vi "封面.vi"() -> ()   [LabVIEW 2013]
uses:
  <vilib>/Utility/config.llb/Config Data RefNum.ctl
  <vilib>/Utility/config.llb/NI_LVConfig.lvlib
panel:
  in  "版本":string
  in  "编号":string
  in  "封面表":T1
  in  "stop":bool
  # "油动机试验报告\nACTUATOR TEST REPORT"
  # "上海汽轮机厂\nSHANGHAI TURBINE PLANT"
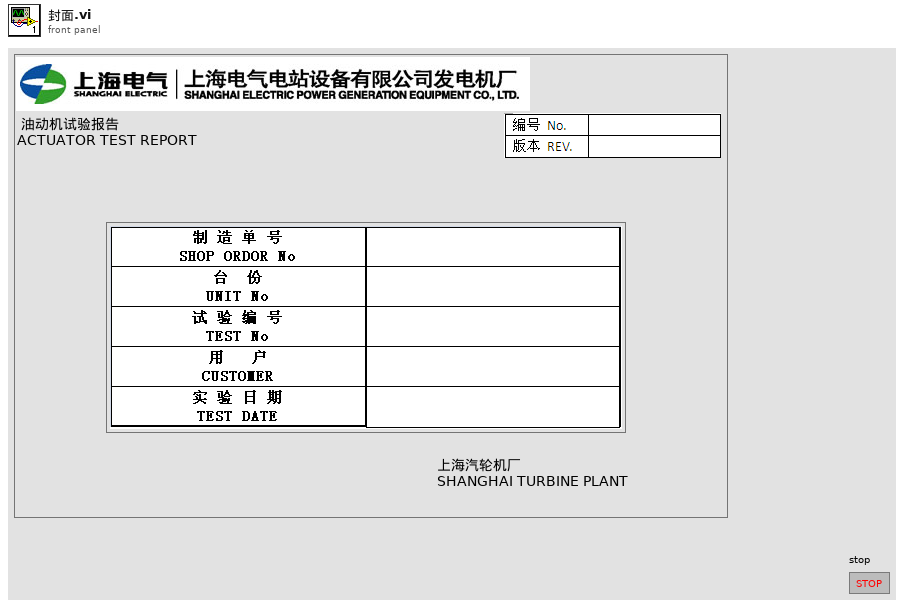
[diagram p1: front panel]
types:
  T1 = typedef "封面表.ctl" = cluster{"制造单号":string, "台份":string, "试验编号":string, "用户":string, "试验日期":string}
  T2 = typedef "NI_LVConfig.lvlib/Config Data RefNum.ctl" = refnum<k1>
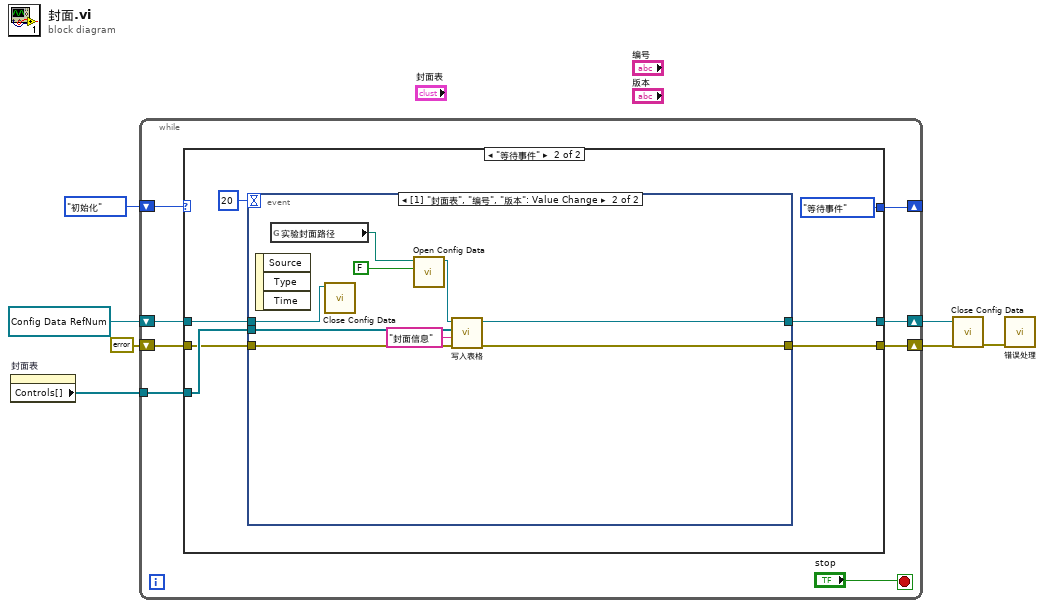
[diagram p0: block diagram]
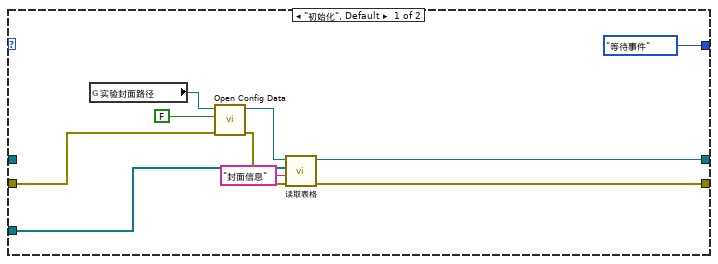
[diagram p2: hidden frame]
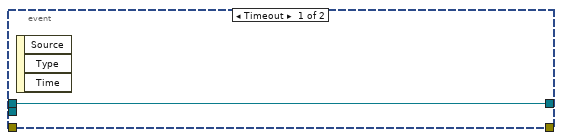
[diagram p3: hidden frame]
diagram:
  w6 = T2 refnum items=["config data"] ("引用句柄输入")
  n1 = property on="封面表" class="Clust (strict)"() -> ("Controls[]"=w5:refnum<vi>[])  [unwired: 2 in, 2 out]
  n2 = while {
    shift-right: [w13] -> _
    shift-left: enum16{"初始化", "等待事件"}."初始化" -> [w14]
    shift-right: [w12] -> w4
    shift-left: w6 -> [w10]
    tunnel: w5 -> [w11]
    shift-right: [w9] -> w3
    shift-left: errorcluster {"status"=FALSE, "code"=0, "source"=""} ("错误输出") -> [w8]
    stop <- "stop" stop-if-true
    n3 = case shown="\"等待事件\"" w14 {
      tunnel: [enum16{"初始化", "等待事件"}."等待事件" enum16{"初始化", "等待事件"}."等待事件"] -> w13
      tunnel: [w22 w28] -> w12
      tunnel: w11 -> [w21 w30]
      tunnel: w10 -> [_ w29]
      tunnel: [w20 w27] -> w9
      tunnel: w8 -> [w18 w26]
      frame "初始化", Default {
        n4 = global read "实验封面路径.vi" "实验封面路径"() -> (w17:path)
        n5 = call <vilib>:"Open Config Data.vi"("error in (no error)"=w18, "create file if necessary (T)"=FALSE, "configuration file path"=w17) -> ("error out"=w19:errorcluster, "refnum"=w24:T2)  [unwired: 6 in, 1 out]
        n6 = call "读取表格.vi"("错误输入"=w19, "section"="封面信息", "Controls[]"=w21, "引用句柄输入"=w24) -> ("错误输出"=w20:errorcluster, "引用句柄输出"=w22:T2)  [unwired: 6 in]
      }
      frame "等待事件" {
        n7 = event shown="[1] \"封面表\", \"编号\", \"版本\": Value Change" {
          selector: _ -> [_ _]
          dyn-events: _ -> [_ _]
          timeout: 20 -> [_ _]
          tunnel: w30 -> [_ w42]
          tunnel: w29 -> [w33 w38]
          tunnel: [w33 w41] -> w28
          tunnel: [_ w40] -> w27
          tunnel: w26 -> [_ w39]
          event Timeout {
            n8 = event-data() -> ()  [unwired: 1 in, 3 out]
          }
          event "编号", "版本": Value Change {
            n9 = event-data() -> ()  [unwired: 1 in, 3 out]
            n10 = global read "实验封面路径.vi" "实验封面路径"() -> (w35:path)
            n11 = call <vilib>:"Close Config Data.vi"("refnum"=w38) -> ()  [unwired: 9 in, 2 out]
            n12 = call <vilib>:"Open Config Data.vi"("create file if necessary (T)"=FALSE, "configuration file path"=w35) -> ("refnum"=w36:T2)  [unwired: 7 in, 2 out]
            n13 = call "写入表格.vi"("error in (no error)"=w39, "section"="封面信息", "Controls[]"=w42, "引用句柄输入"=w36) -> ("错误输出"=w40:errorcluster, "引用句柄输出"=w41:T2)  [unwired: 6 in]
          }
        }
      }
    }
  }
  n14 = call <vilib>:"Close Config Data.vi"("error in (no error)"=w3, "refnum"=w4) -> ("error out"=w1:errorcluster)  [unwired: 8 in, 1 out]
  n15 = call "错误处理.vi"("error in (no error)"=w1) -> ()  [unwired: 2 in]
